vi "Handle Relinquish Request.vi"(8 "error in (no error)":errorcluster, 11 "RDS Controller Actor in":refnum<class "RDS Controller Actor.lvclass">) -> (0 "error out":errorcluster, 3 "RDS Controller Actor out":refnum<class "RDS Controller Actor.lvclass">)   [LabVIEW 2015, in "RDS Controller Actor.lvlib" / "RDS Controller Actor.lvclass"]
uses:
  RDS Controller Actor.lvclass
  Controller.ctl
  Libraries/RDS Child Messages/Controller Message/Controller Message.lvclass
  Libraries/RDS Framework/RDS Message ID.ctl
  Libraries/RDS Child Messages/Controller Message/Controller Message Type.ctl
  Libraries/RDS Framework/RDS Message Class/RDS Message.lvclass/RDS Message.ctl
  Libraries/RDS Child Messages/Controller Message/Controller Message.lvclass/Controller Message.ctl
  RDS Controller Actor.lvclass/RDS Controller Actor.ctl
  Libraries/RDS Child Messages/RDS Child Messages.lvlib
  Libraries/RDS Framework/RDS Message Class/RDS Message.lvclass
  RDS Parent Actor/RDS Parent Actor/RDS Parent Actor.lvclass
  RDS Helm Actor/RDS Helm Actor.lvlib
  RDS Controller Actor.lvlib
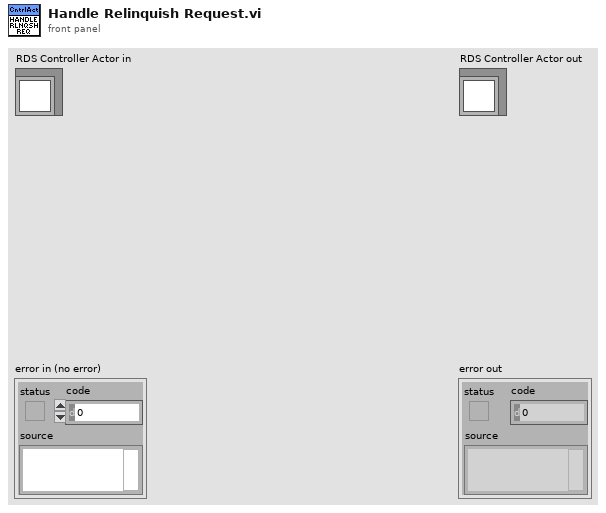
[diagram p1: front panel]
types:
  T1 = typedef "RDS Controller Actor.lvlib/Controller.ctl" = enum16{"Idle", "Local Remote Control", "Shore Remote Control", "Mission Control"}
  T2 = typedef "RDS Child Messages.lvlib/Controller Message.lvclass/Controller Message Type.ctl" = enum16{"Control Relinquish Request", "Control Relinquish Command", "Control Request", "Control Granted"}
  T3 = typedef "RDS Child Messages.lvlib/RDS Message ID.ctl" = enum16{"RDS Hello World", "String Message", "AIP_Status", "AIP_Command", "GPS_Data", "MCB_Command", "MCB_Status", "Compass_Data", "Depth_Data", "Battery_Data", "Contoller_State", "Set_Mag_Dev", "BTB_Shutdown", "State_Sample_Request", "State_Sample", "PID_Gains_Set", "Helm_Limiter_Set", "Helm_Heading_Command", "Helm_Steering_Command", "Helm_Status", "Controller_Message", "AIP_Set_Min_Depth", "Mission_Controller_State", "Mission_Upload", "Mission_Set_Op_and_Run", "Mission_Settings_Set"}
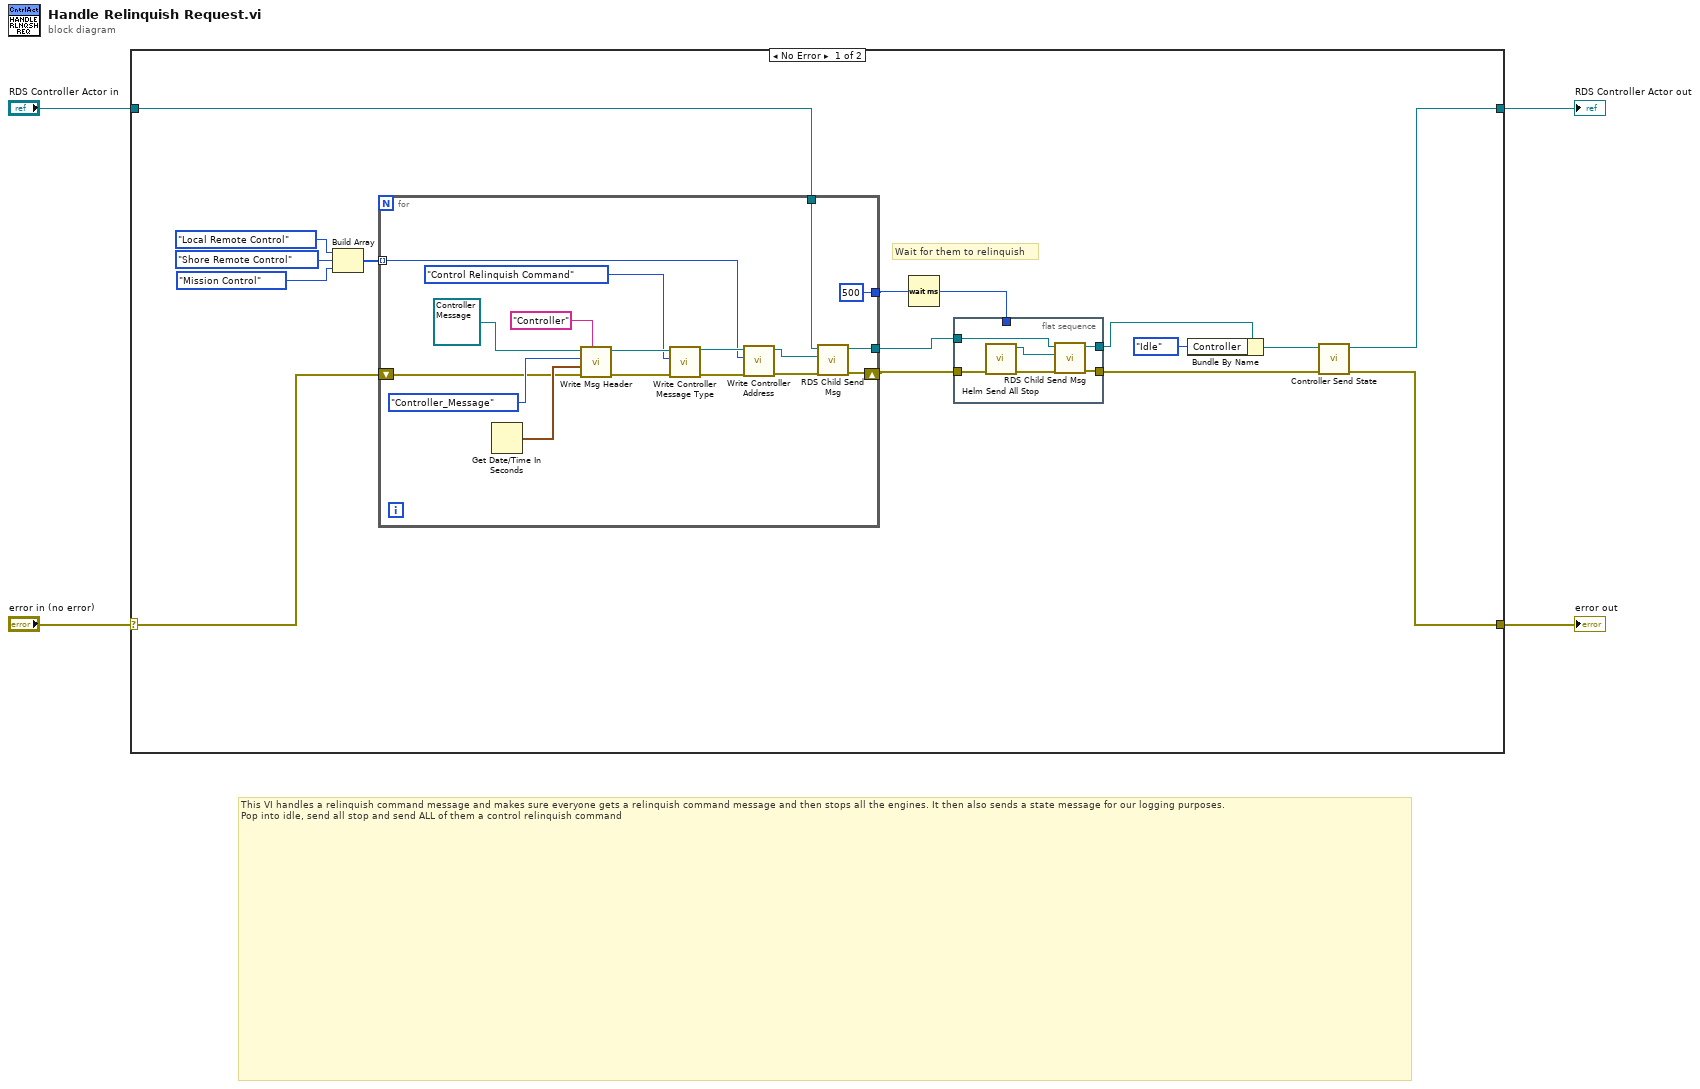
[diagram p0: block diagram]
diagram:
  # "This VI handles a relinquish command message and makes sure everyone gets a relinquish command message and then stops all the engines. It then also sends a state message for our logging purposes.\nPop into idle, send all stop and send ALL of them a control relinquish command"
  n1 = case shown="No Error" "error in (no error)" {
    selector: "error in (no error)" -> [w11 w45]
    tunnel: [w7 w45] -> w3
    tunnel: [w6 w44] -> w1
    tunnel: "RDS Controller Actor in" -> [w16 w44]
    frame No Error {
      # "Wait for them to relinquish"
      n2 = Build Array(Controller."Local Remote Control" ("Current Controller"), Controller."Shore Remote Control" ("Current Controller"), Controller."Mission Control" ("Current Controller")) -> (w20:T1[])
      n3 = for {
        tunnel: w20 -> [w35] mode=indexing
        tunnel: w16 -> [w32]
        tunnel: [u32 500 ("milliseconds to wait")] -> w18
        shift-right: [w31] -> w17
        shift-left: w11 -> [w28]
        tunnel: [w27] -> w5
        n4 = Get Date/Time In Seconds() -> (seconds since 1Jan1904=w40:timestamp)
        n5 = call "Write Msg Header.vi"("Sender Name"="Controller", "error in (no error)"=w28, "Time Stamp"=w40, "Msg ID"=RDS_Message_ID."Controller_Message", "RDS Message in"=refnum<class "Controller Message.lvclass"> refnum ("RDS Child Messages.lvlib:Controller Message.lvclass")) -> ("error out"=w39:errorcluster, "RDS Message out"=w38:refnum<class "Controller Message.lvclass">)  [unwired: 5 in]
        n6 = call "Write Controller Message Type.vi"("error in (no error)"=w39, "Controller Message Type"=Controller_Message_Type."Control Relinquish Command", "Controller Message in"=w38) -> ("error out"=w34:errorcluster, "Controller Message out"=w36:refnum<class "Controller Message.lvclass">)  [unwired: 7 in]
        n7 = call "Write Controller Address.vi"("error in (no error)"=w34, "Controller"=w35, "Controller Message in"=w36) -> ("error out"=w33:errorcluster, "Controller Message out"=w29:refnum<class "Controller Message.lvclass">)  [unwired: 7 in]
        n8 = call "RDS Child Send Msg.vi"("error in (no error)"=w33, "RDS Message"=w29, "RDS Parent Actor in"=w32) -> ("error out"=w31:errorcluster, "RDS Parent Actor out"=w27:refnum<class "RDS Controller Actor.lvclass">)  [unwired: 7 in]
      }
      n9 = Wait (ms)(milliseconds to wait=w18) -> (millisecond timer value=w19:u32)
      n10 = flat-sequence {
        tunnel: w17 -> [w26]
        tunnel: w19 -> [_]
        tunnel: [w24] -> w8
        tunnel: [w22] -> w10
        tunnel: w5 -> [w21]
        frame #0 {
          n11 = call "Helm Send All Stop.vi"("error in (no error)"=w26) -> ("error out"=w25:errorcluster, "All Stop Message"=w23:refnum<class "Steering Command.lvclass">)  [unwired: 9 in]
          n12 = call "RDS Child Send Msg.vi"("error in (no error)"=w25, "RDS Message"=w23, "RDS Parent Actor in"=w21) -> ("error out"=w24:errorcluster, "RDS Parent Actor out"=w22:refnum<class "RDS Controller Actor.lvclass">)  [unwired: 7 in]
        }
      }
      n13 = Bundle By Name(cluster=w10, "Controller"=Controller."Idle") -> (w9:refnum<class "RDS Controller Actor.lvclass">)
      n14 = call "Controller Send State.vi"("error in (no error)"=w8, "RDS Controller Actor in"=w9) -> ("error out"=w7:errorcluster, "RDS Controller Actor out"=w6:refnum<class "RDS Controller Actor.lvclass">)  [unwired: 8 in]
    }
    frame Error {
    }
  }
  "error out" <- w3
  "RDS Controller Actor out" <- w1
